vi "Main Page.vi"(8 "error in (no error)":errorcluster, 11 "Node Ptr":T1 format="%.0x") -> (0 "error out":errorcluster)   [LabVIEW 2027, in "System Monitor System Explorer.lvlib"]
uses:
  System Monitor System Explorer.lvlib
  <vilib>/NI VeriStand/Custom Device API/Custom Device Item Ref.ctl
  <vilib>/NI VeriStand/Custom Device API/Custom Device API.lvlib
panel:
  in  "Number of CPU Cores":u64=4 min=1 max=1000 step=1
  in  "Update Rate (Hz)":dbl=10.0 min=1e-06 max=1000.0 step=1.0
  in  "SHDocVw.IWebBrowser":refnum<k7>(container)
  in  "Specific Header":cluster{"Section Name":string}={"Section Name"="Custom Device Item Settings"}
  in  "General Header":cluster{"Section Name":string}={"Section Name"="General Custom Device Settings"}
  in  "Description":string
  in  "Name":string
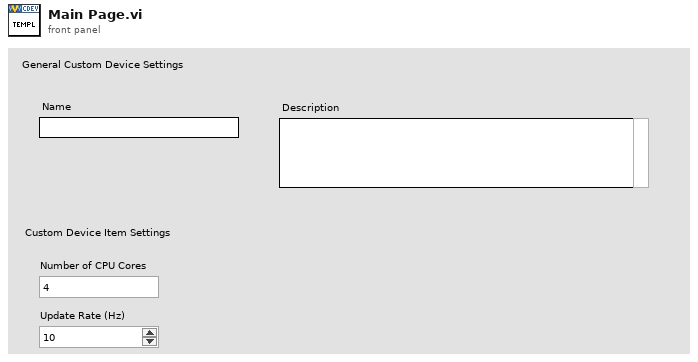
[diagram p1: front panel]
types:
  T1 = typedef "Custom Device API.lvlib/Custom Device Item Ref.ctl" = u64
  T2 = typedef "Custom Device API.lvlib/Custom Device Item Info.ctl" = cluster{"Name":string, "Is Channel":bool, "GUID":string, "Is Waveform":bool}
  T3 = typedef "System Monitor Shared.lvlib/System Monitor Settings.ctl" = cluster{"Number of CPU Cores":u64, "Update Rate (Hz)":dbl}
  T4 = typedef "Custom Device API.lvlib/Custom Device Commands.ctl" = enum16{"Default", "Item renamed", "Shutdown", "Dynamic button pressed"}
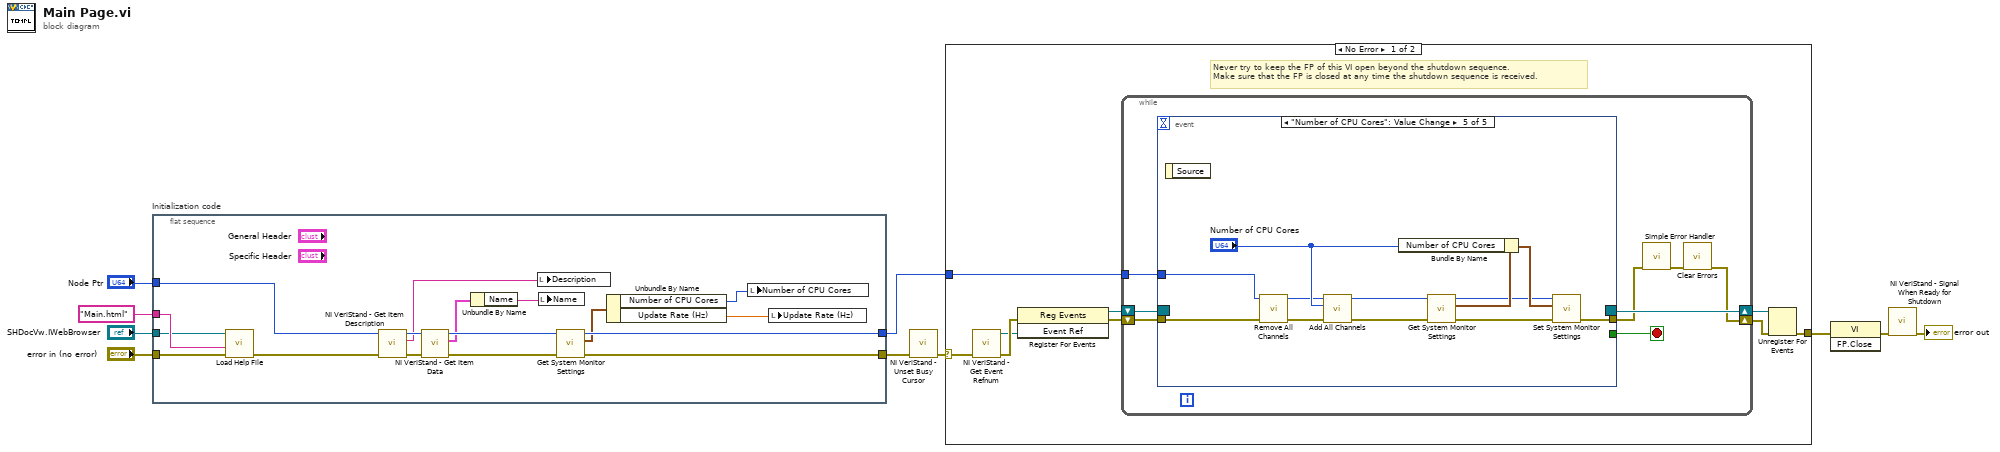
[diagram p0: block diagram]
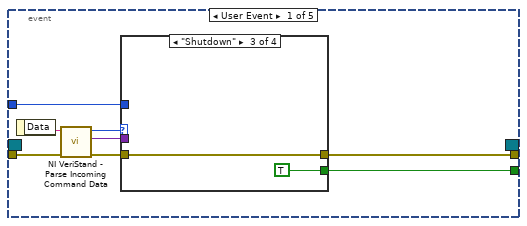
[diagram p2: hidden frame]
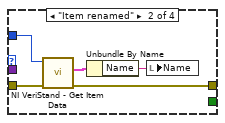
[diagram p4: hidden frame]
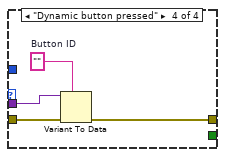
[diagram p5: hidden frame]
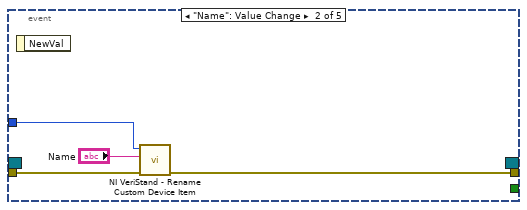
[diagram p6: hidden frame]
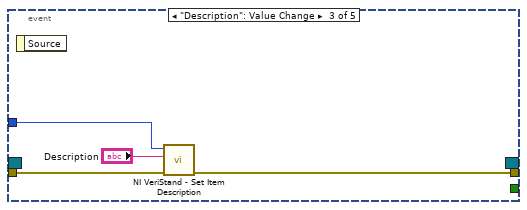
[diagram p7: hidden frame]
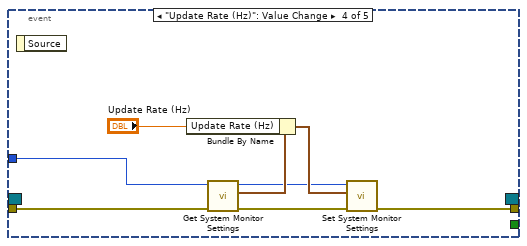
[diagram p8: hidden frame]
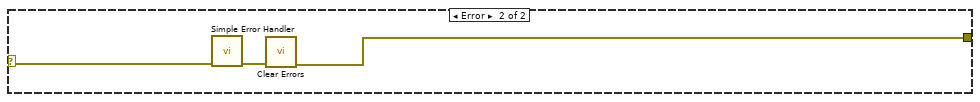
[diagram p9: hidden frame]
diagram:
  n1 = flat-sequence "Initialization code" {
    tunnel: "error in (no error)" -> [w23]
    tunnel: "Node Ptr" -> [w12]
    tunnel: [w16] -> w6
    tunnel: [w18] -> w3
    tunnel: "SHDocVw.IWebBrowser" -> [w21]
    tunnel: "Main.html" ("HTML File") -> [w22]
    frame #0 {
      n2 = call "Load Help File.vi"("error in (no error)"=w23, "HTML File to Load"=w22, "Browser"=w21) -> ("error out"=w11:errorcluster)  [unwired: 8 in]
      n3 = call <vilib>:"NI VeriStand - Get Item Description.vi"("error in (no error)"=w11, "Item Ref in"=w12) -> ("error out"=w25:errorcluster, "Description"=w19:string, "Item Ref out"=w26:T1)  [unwired: 7 out]
      n4 = call <vilib>:"NI VeriStand - Get Item Data.vi"("error in (no error)"=w25, "Item Ref in"=w26) -> ("error out"=w17:errorcluster, "Item Info"=w24:T2, "Item Ref out"=w27:T1)  [unwired: 7 out]
      n5 = Unbundle By Name(w24) -> ("Name"=w20:string)
      n6 = local write "Description"(w19) -> ()
      n7 = local write "Name"(w20) -> ()
      n8 = call "Get System Monitor Settings.vi"("error in (no error)"=w17, "Item Ref in"=w27) -> ("error out"=w16:errorcluster, "System Monitor Settings"=w15:T3, "Item Ref out"=w18:T1)  [unwired: 7 in]
      n9 = Unbundle By Name(w15) -> ("Number of CPU Cores"=w13:u64, "Update Rate (Hz)"=w14:dbl)
      n10 = local write "Number of CPU Cores"(w13) -> ()
      n11 = local write "Update Rate (Hz)"(w14) -> ()
    }
  }
  n12 = call <vilib>:"NI VeriStand - Unset Busy Cursor.vi"("error in (no error)"=w6) -> ("error out"=w5:errorcluster)  [unwired: 10 out]
  n13 = case shown="No Error" w5 {
    selector: w5 -> [w28 w95]
    tunnel: [w33 w93] -> w10
    tunnel: w3 -> [w29 _]
    frame No Error {
      # "Never try to keep the FP of this VI open beyond the shutdown sequence.\nMake sure that the FP is closed at any time the shutdown sequence is received."
      n14 = call <vilib>:"NI VeriStand - Get Event Refnum.vi"("error in (no error)"=w28) -> ("error out"=w36:errorcluster, "Event Ref"=w32:refnum<user-event>)  [unwired: 9 out]
      n15 = register-events(error in=w36, w32) -> (reference out=w30:refnum<event-registration>, error out=w31:errorcluster)  [unwired: 1 in]
      n16 = while {
        tunnel: w29 -> [w40]
        shift-right: [w37] -> w34
        shift-left: w31 -> [w43]
        shift-right: [w44] -> w35
        shift-left: w30 -> [w42]
        stop <- w41 stop-if-true
        n17 = event shown="[4] \"Number of CPU Cores\": Value Change" {
          selector: w42 -> [_ _ _ _ _]
          dyn-events: [_ _ _ _ _] -> w44
          timeout: _ -> [_ _ _ _ _]
          tunnel: w43 -> [w52 w68 w71 w80 w87]
          tunnel: [w48 _ _ _ _] -> w41
          tunnel: [w47 w67 w70 w76 w88] -> w39
          tunnel: w40 -> [w46 w66 w72 w78 w86]
          event User Event {
            n18 = event-data() -> ("Data"=w51:string)  [unwired: 1 out]
            n19 = call <vilib>:"NI VeriStand - Parse Incoming Command Data.vi"("error in (no error)"=w52, "Incoming data"=w51) -> ("error out"=w50:errorcluster, "Outgoing data"=w45:variant, "Action"=w49:T4)  [unwired: 7 out]
            n20 = case shown="\"Shutdown\"" w49 {
              tunnel: w50 -> [w53 w58 w59 w64]
              tunnel: [_ _ TRUE _] -> w48
              tunnel: [w53 w55 w59 w61] -> w47
              tunnel: w46 -> [_ w57 _ _]
              tunnel: w45 -> [_ _ _ w63]
              frame "Default", Default {
              }
              frame "Item renamed" {
                n21 = call <vilib>:"NI VeriStand - Get Item Data.vi"("error in (no error)"=w58, "Item Ref in"=w57) -> ("error out"=w55:errorcluster, "Item Info"=w56:T2)  [unwired: 8 out]
                n22 = Unbundle By Name(w56) -> ("Name"=w54:string)
                n23 = local write "Name"(w54) -> ()
              }
              frame "Shutdown" {
              }
              frame "Dynamic button pressed" {
                w62 = ""  # Button ID
                n24 = Variant To Data(error in=w64, type=w62, Variant=w63) -> (error out=w61:errorcluster)  [unwired: 1 out]
              }
            }
          }
          event "Name": Value Change {
            n25 = event-data() -> ()  [unwired: 2 out]
            n26 = call <vilib>:"NI VeriStand - Rename Custom Device Item.vi"("error in (no error)"=w68, "New Name"="Name", "Item Ref in"=w66) -> ("error out"=w67:errorcluster)  [unwired: 1 in, 7 out]
          }
          event "Description": Value Change {
            n27 = event-data() -> ()  [unwired: 2 out]
            n28 = call <vilib>:"NI VeriStand - Set Item Description.vi"("error in (no error)"=w71, "Description"="Description", "Item Ref in"=w72) -> ("error out"=w70:errorcluster)  [unwired: 8 out]
          }
          event "Update Rate (Hz)": Value Change {
            n29 = event-data() -> ()  [unwired: 2 out]
            n30 = call "Get System Monitor Settings.vi"("error in (no error)"=w80, "Item Ref in"=w78) -> ("error out"=w79:errorcluster, "System Monitor Settings"=w77:T3, "Item Ref out"=w74:T1)  [unwired: 7 in]
            n31 = Bundle By Name(cluster=w77, "Update Rate (Hz)"="Update Rate (Hz)") -> (w75:T3)
            n32 = call "Set System Monitor Settings.vi"("error in (no error)"=w79, "System Monitor Settings"=w75, "Item Ref in"=w74) -> ("error out"=w76:errorcluster)  [unwired: 7 in, 1 out]
          }
          event "Number of CPU Cores": Value Change {
            n33 = event-data() -> ()  [unwired: 2 out]
            n34 = call "Remove All Channels.vi"("error in (no error)"=w87, "Item Ref in"=w86) -> ("error out"=w85:errorcluster, "Item Ref out"=w83:T1)  [unwired: 8 in]
            n35 = call "Add All Channels.vi"("error in (no error)"=w85, "Number of CPU Cores in"="Number of CPU Cores", "Item Ref in"=w83) -> ("error out"=w81:errorcluster, "Item Ref out"=w82:T1)  [unwired: 7 in]
            n36 = call "Get System Monitor Settings.vi"("error in (no error)"=w81, "Item Ref in"=w82) -> ("error out"=w92:errorcluster, "System Monitor Settings"=w91:T3, "Item Ref out"=w89:T1)  [unwired: 7 in]
            n37 = Bundle By Name(cluster=w91, "Number of CPU Cores"="Number of CPU Cores") -> (w90:T3)
            n38 = call "Set System Monitor Settings.vi"("error in (no error)"=w92, "System Monitor Settings"=w90, "Item Ref in"=w89) -> ("error out"=w88:errorcluster)  [unwired: 7 in, 1 out]
          }
        }
        n39 = call <vilib>:"Simple Error Handler.vi"("error in (no error)"=w39) -> ("error out"=w38:errorcluster)  [unwired: 1 in, 7 out]
        n40 = call <vilib>:"Clear Errors.vi"("error in (no error)"=w38) -> ("error out"=w37:errorcluster)  [unwired: 1 in, 5 out]
      }
      n41 = Unregister For Events(event registration refnum=w35, error in=w34) -> (error out=w33:errorcluster)
    }
    frame Error {
      n42 = call <vilib>:"Simple Error Handler.vi"("error in (no error)"=w95) -> ("error out"=w94:errorcluster)  [unwired: 1 in, 7 out]
      n43 = call <vilib>:"Clear Errors.vi"("error in (no error)"=w94) -> ("error out"=w93:errorcluster)  [unwired: 1 in, 5 out]
    }
  }
  n44 = invoke class="VI" method="FP.Close"(error in=w10) -> (error out=w9:errorcluster)  [unwired: 2 in, 2 out]
  n45 = call <vilib>:"NI VeriStand - Signal When Ready for Shutdown.vi"("error in (no error)"=w9) -> ("error out"=→"error out":errorcluster)  [unwired: 10 out]
